vi "PointerArray_Offset.vi"(7 "Buffer":T1, 10 "Total Starting Offset":i32, 11 "Pointer Array":refnum<class "((Pointer)).lvclass">[](array[class])) -> (3 "Pointer Array Out":refnum<class "((Pointer)).lvclass">[](array[class]))   [LabVIEW 2016, in "(WavBuf).lvclass"]
uses:
  WavBuf/(WavBuf).lvclass
  Pointer/((Pointer)).lvclass
  TypeDefs_Utility/Ref_DVR_Buffer.ctl
  Universal Controls/Waveform_Data.ctl
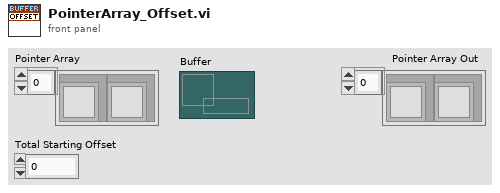
[diagram p1: front panel]
types:
  T1 = typedef "Ref_DVR_Buffer.ctl" = refnum<data-value>
  T2 = typedef "Waveform_Data.ctl" = waveform(dbl)
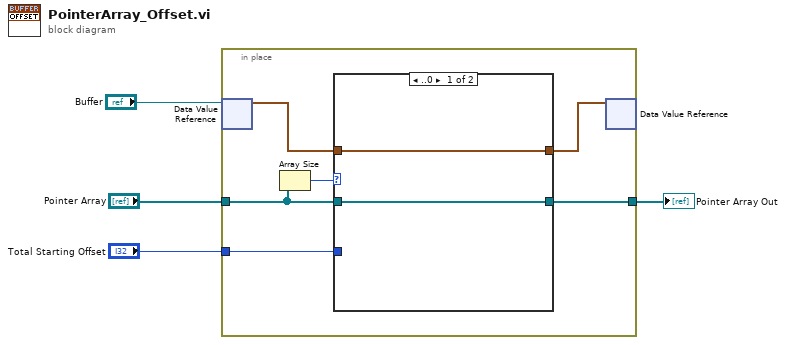
[diagram p0: block diagram]
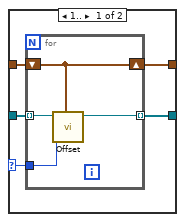
[diagram p3: hidden frame]
diagram:
  n1 = in-place {
    in-place-border: [w10] -> w4
    in-place-border: "Total Starting Offset" -> [w9]
    in-place-border: "Pointer Array" -> [w8]
    n2 = in-place-dvr #1("Buffer") -> (w6:T2)  [unwired: 1 out]
    n3 = Array Size(array=w8) -> (size(s)=w7:i32)
    n4 = case shown="..0" w7 {
      tunnel: [w12 w17] -> w10
      tunnel: w9 -> [_ w16]
      tunnel: w8 -> [w12 w15]
      tunnel: w6 -> [w11 w14]
      tunnel: [w11 w13] -> w5
      frame ..0 {
      }
      frame 1.. {
        n5 = case shown="..0" w16 {
          selector: w16 -> [w22 _]
          tunnel: w15 -> [w21 w28]
          tunnel: [w20 w28] -> w17
          tunnel: w14 -> [w19 w27]
          tunnel: [w18 w27] -> w13
          frame 1.. {
            n6 = for {
              tunnel: w22 -> [w24]
              tunnel: w21 -> [w26] mode=indexing
              tunnel: [w25] -> w20 mode=indexing
              shift-right: [w23] -> w18
              shift-left: w19 -> [w23]
              n7 = call-dynamic "Offset.vi"("Raw Data Waveform"=w23, "Offset"=w24, "((Pointer))"=w26) -> ("((Pointer)) Out"=w25:refnum<class "((Pointer)).lvclass">)  [unwired: 8 in]
            }
          }
          frame ..0 {
          }
        }
      }
    }
    n8 = in-place-dvr #1(w5) -> ()  [unwired: 2 out]
  }
  "Pointer Array Out" <- w4
